vi "TimestampMsToString.vi"(11 "timestamp_ms":i64) -> (3 "timestamp_str":string)   [LabVIEW 2026]
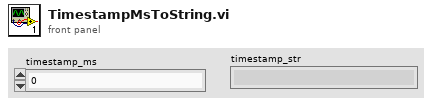
[diagram p1: front panel]
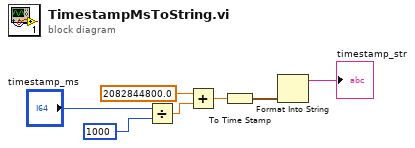
[diagram p0: block diagram]
diagram:
  n1 = Divide(x="timestamp_ms", y=1000) -> (x/y=w3:dbl)
  n2 = Add(x=2082844800.0, y=w3) -> (x+y=w1:dbl)
  n3 = To Time Stamp(1:w1) -> (0:w7:timestamp)
  n4 = Format Into String(w7) -> (resulting string=→"timestamp_str":string)  [unwired: 3 in, 1 out]
